vi "Message for Generation.vi"(8 "Error In":errorcluster, 11 "eHS Core Index":T1) -> (0 "Error Out":errorcluster, 3 "Message":string)   [LabVIEW 2017]
uses:
  <vilib>/OPAL-RT/eHS Toolkit/eHS Matrix Generation/_Controls/eHS Core Index.ctl
  <vilib>/OPAL-RT/eHS Toolkit/eHS Matrix Generation/eHS Matrix Generation.lvlib
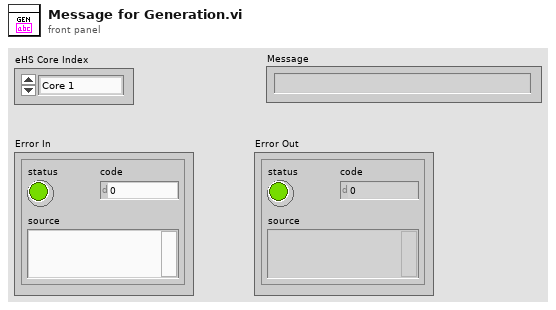
[diagram p1: front panel]
types:
  T1 = typedef "OPAL-RT eHS.lvlib/eHS Matrix Generation.lvlib/eHS Core Index.ctl" = enum16{"Core 1", "Core 2", "Core 3", "Core 4", "Core 5", "Core 6", "Core 7", "Core 8", "Core 9", "Core 10"}
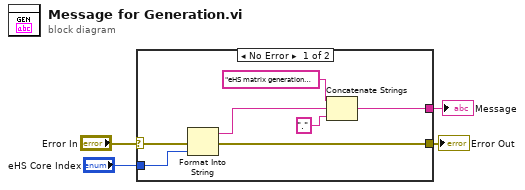
[diagram p0: block diagram]
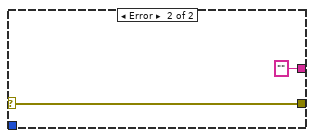
[diagram p2: hidden frame]
diagram:
  n1 = case shown="No Error" "Error In" {
    selector: "Error In" -> [w11 w13]
    tunnel: [w5 w13] -> w3
    tunnel: "eHS Core Index" -> [w10 _]
    tunnel: [w6 ""] -> w1
    frame No Error {
      n2 = Format Into String(error in=w11, w10) -> (resulting string=w9:string, error out=w5:errorcluster)  [unwired: 2 in]
      n3 = Concatenate Strings("eHS matrix generation complete for ", w9, ".") -> (w6:string)
    }
    frame Error {
    }
  }
  "Error Out" <- w3
  "Message" <- w1
